vi "SLAVEOF-HOSTPORT.vi"(0 "refnum in":refnum<vi>, 5 "Host":string, 7 "Port":string, 11 "error in":errorcluster) -> (4 "refnum out":refnum<vi>, 6 "Data":T1, 15 "error out":errorcluster)   [LabVIEW 2020]
uses:
  SubVIs/Controls/redis-data.ctl
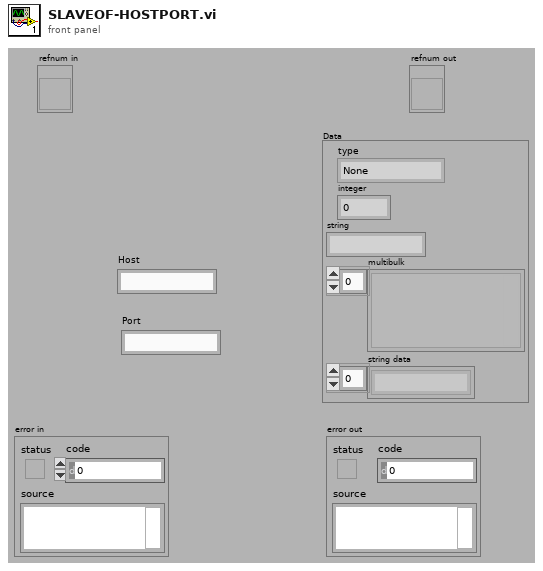
[diagram p1: front panel]
types:
  T1 = typedef "redis-data.ctl" = cluster{"type":enum16{"None", "Error", "Status", "Nil", "Integer", "String", "Multibulk"}, "integer":i64, "string":string, "multibulk":variant[], "string data":string[]}
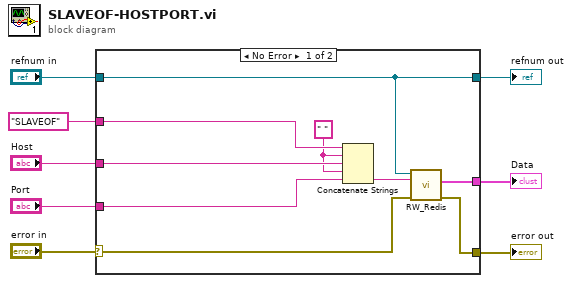
[diagram p0: block diagram]
diagram:
  n1 = case shown="No Error" "error in" {
    selector: "error in" -> [w15 w19]
    tunnel: "Host" -> [w12 _]
    tunnel: "SLAVEOF" -> [w17 _]
    tunnel: "refnum in" -> [w10 w18]
    tunnel: [w14 w19] -> w6
    tunnel: [w13 _] -> w1
    tunnel: "Port" -> [w11 _]
    tunnel: [w10 w18] -> w2
    frame No Error {
      w9 = " "
      n2 = Concatenate Strings(w17, w9, w12, w9, w11) -> (w16:string)
      n3 = call "RW_Redis.vi"("error in"=w15, "command"=w16, "refnum"=w10) -> ("error out"=w14:errorcluster, "Data"=w13:T1)  [unwired: 7 in]
    }
    frame Error {
    }
  }
  "error out" <- w6
  "refnum out" <- w2
  "Data" <- w1
